vi "PmodMIC3Read.vi"(5 "CS Channel":u8, 7 "SPI Channel (0)":u8, 8 "error in (no error)":errorcluster, 10 "Supply Voltage":dbl, 11 "LINX Resource in":T1) -> (0 "error out":errorcluster, 2 "Voltage (V)":dbl, 3 "LINX Resource out":T1)   [LabVIEW 2014]
doc: "Read the specified SPI channel. SPI is full duplex, therefore the write and read operations take place simultaneously.\n\nSPI Channel: specifies the device SPI channel to write/read to.\n\nThis VI outputs the voltage reading from the MIC3.\n\nCS Channel: the Chip Select (DIO) channel to use during the SPI transaction. The default channel is 10.\n\nCS Logic Level: specifies the logic level of the CS pin. Active low is most common and means that CS will idle high, then be driven low when a frame begins. All Data bytes are shifted out, then CS will be driven high to end the frame. PmodMIC3 is active low."
uses:
  <vilib>/MakerHub/LINX/Private/Type Defs/LINX Ref.ctl
  <vilib>/MakerHub/LINX/Private/Type Defs/Platform.ctl
  <vilib>/MakerHub/LINX/Private/Type Defs/Interface.ctl
  <vilib>/MakerHub/LINX/Private/Device/Type Defs/LINX Device Config.ctl
  <vilib>/MakerHub/LINX/Private/Device/Type Defs/TCP Config.ctl
  <vilib>/MakerHub/LINX/Private/Device/Type Defs/Channels.ctl
  <vilib>/MakerHub/LINX/Public/Peripherals/SPI/SPI CS Config.ctl
  <vilib>/MakerHub/LINX/Private/Type Defs/Peripherals/SPI/SPI CS Logic Level.ctl
  <vilib>/MakerHub/LINX/Public/Peripherals/SPI/SPI Write Read 1 Frame.vi
  <vilib>/MakerHub/LINX/LMH-LINX.lvlib
  <vilib>/MakerHub/LINX/Private/Device/Device.lvlib
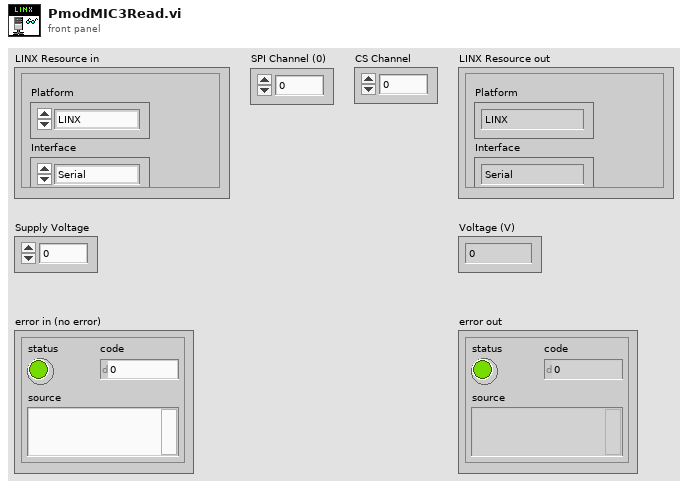
[diagram p1: front panel]
types:
  T1 = typedef "LMH-LINX.lvlib/LINX Ref.ctl" = cluster{"Platform":T2, "Interface":T3, "LINX Device Config":T4}
  T2 = typedef "LMH-LINX.lvlib/Platform.ctl" = enum16{"LINX", "myRIO"}
  T3 = typedef "LMH-LINX.lvlib/Interface.ctl" = enum16{"Serial", "TCP"}
  T4 = typedef "LMH-LINX.lvlib/Device.lvlib/LINX Device Config.ctl" = cluster{"Interface":T3, "COM Port":refnum<visa-resource-name>, "TCP Configuration":T5, "Device Family":u8, "Device ID":u8, "Device Name":string, "TCP Ref":refnum<k5>, "Channels":T6}
  T5 = typedef "LMH-LINX.lvlib/Device.lvlib/TCP Config.ctl" = cluster{"IP Address":string, "Port":u16}
  T6 = typedef "LMH-LINX.lvlib/Channels.ctl" = cluster{"DI":u8[], "DO":u8[], "AI":u8[], "AO":u8[], "PWM":u8[], "QE":u8[], "UART":u8[], "I2C 2":u8[], "SPI":u8[], "CAN":u8[], "Servo":u8[], "AI Ref (V)":dbl, "AO Ref (V)":dbl, "AO Resolution (Bits)":u8}
  T7 = typedef "LMH-LINX.lvlib/SPI CS Config.ctl" = cluster{"CS Channel":u8, "CS Logic Level":T8}
  T8 = typedef "LMH-LINX.lvlib/SPI CS Logic Level.ctl" = enum8{"Active Low", "Active High"}
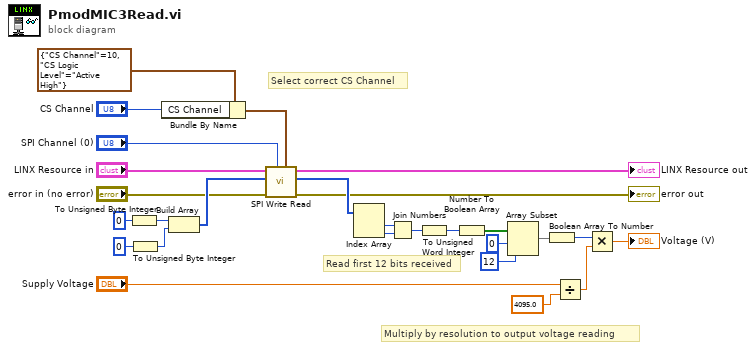
[diagram p0: block diagram]
diagram:
  # "Multiply by resolution to output voltage reading"
  # "Read first 12 bits received"
  # "Select correct CS Channel"
  n1 = To Unsigned Byte Integer(number=0) -> (unsigned 8bit integer=w10:u8)
  n2 = To Unsigned Byte Integer(number=0) -> (unsigned 8bit integer=w9:u8)
  n3 = Bundle By Name(cluster=T7 {"CS Channel"=10, "CS Logic Level"=enum."Active High"} ("CS Configuration"), "CS Channel"="CS Channel") -> (w1:T7)
  n4 = Build Array(w10, w9) -> (w11:u8[])
  n5 = call-poly <vilib>:"SPI Write Read.vi"("CS Configuration"=w1, "SPI Channel (0)"="SPI Channel (0)", "Error In"="error in (no error)", "Data"=w11, "LINX Resource"="LINX Resource in") -> ("Error Out"=→"error out":errorcluster, "Read Data"=w20:u8[], "LINX Resource"=→"LINX Resource out":T1)  [unwired: 4 in]
  n6 = Index Array(array=w20) -> (element #1=w13:u8, element #2=w14:u8)  [unwired: 2 in]
  n7 = Join Numbers(hi=w13, lo=w14) -> ((hi.lo)=w12:u16)
  n8 = To Unsigned Word Integer(number=w12) -> (unsigned 16bit integer=w15:u16)
  n9 = Number To Boolean Array(number=w15) -> (Boolean array=w16:bool[])
  n10 = Array Subset(array=w16, index=0, length=12) -> (w19:bool[])
  n11 = Boolean Array To Number(Boolean array=w19) -> (number=w21:u16)
  n12 = Divide(x="Supply Voltage", y=4095.0) -> (x/y=w24:dbl)
  n13 = Multiply(x=w21, y=w24) -> (x*y=→"Voltage (V)":dbl)
